vi "GetLidarDistance.vi"(8 "error in":errorcluster, 11 "Channel Name":tag="A/I2C") -> (0 "error out":errorcluster, 3 "(hi.lo)":u16)   [LabVIEW 2017]
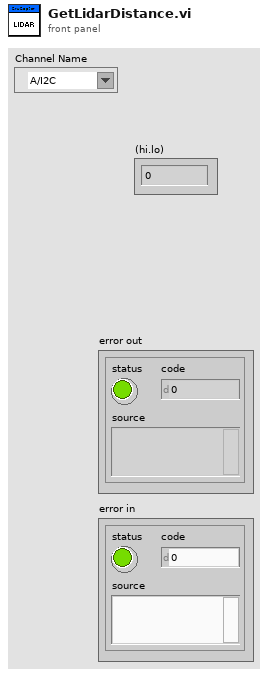
[diagram p1: front panel]
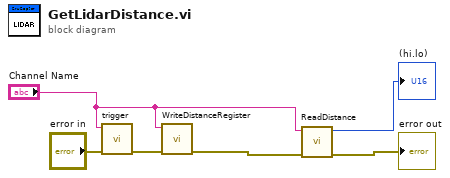
[diagram p0: block diagram]
diagram:
  n1 = call "trigger.vi"("error in (no error)"="error in", "Channel Name"="Channel Name") -> ("error out"=w6:errorcluster)  [unwired: 9 in]
  n2 = call "WriteDistanceRegister.vi"("error in (no error)"=w6, "Channel Name"="Channel Name") -> ("error out"=w5:errorcluster)  [unwired: 9 in]
  n3 = call "ReadDistance.vi"("error in (no error)"=w5, "Channel Name"="Channel Name") -> ("error out"=→"error out":errorcluster, "(hi.lo)"=→"(hi.lo)":u16)  [unwired: 8 in]
